vi "Monitoring task.vi"   [LabVIEW 2016]
types:
  T1 = cluster{bool, "测试模式":enum16{"水样测试", "平行样测试", "集成干预测试", "加标回收"}}
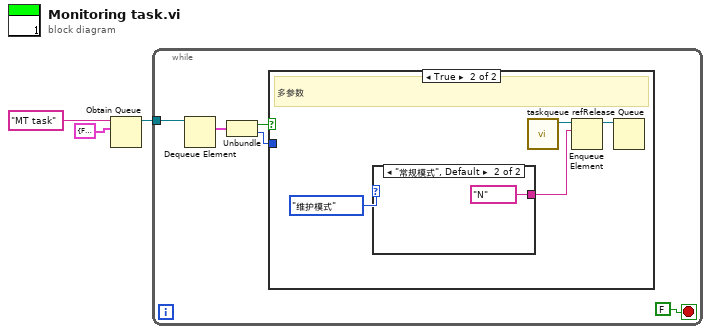
[diagram p0: block diagram]
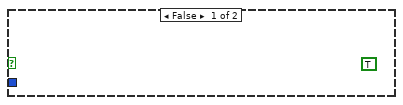
[diagram p2: hidden frame]
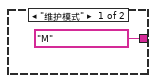
[diagram p3: hidden frame]
diagram:
  n1 = Obtain Queue(name (unnamed)="MT task" ("名称（未命名）"), element data type=T1 {FALSE, "测试模式"=enum."水样测试"}) -> (queue out=w2:refnum<queue>)  [unwired: 3 in, 2 out]
  n2 = while {
    tunnel: w2 -> [w8]
    stop <- FALSE stop-if-true
    n3 = Dequeue Element(queue=w8) -> (element=w6:T1)  [unwired: 2 in, 3 out]
    n4 = Unbundle(w6) -> (w5:bool, "测试模式"=w4:enum16{"水样测试", "平行样测试", "集成干预测试", "加标回收"})
    n5 = case shown="True" w5 {
      tunnel: w4 -> [_ _]
      frame False {
        (unwired) TRUE ("t")
      }
      frame True {
        # "多参数"
        n6 = case shown="\"常规模式\", Default" enum16{"维护模式", "常规模式", "应急模式", "质控模式"}."维护模式" ("运行模式") {
          tunnel: ["M" ("数据标记表") "N" ("数据标记表")] -> w12
          frame "维护模式" {
          }
          frame "常规模式", Default {
          }
        }
        n7 = call "taskqueue ref.vi"() -> ("队列输出"=w11:refnum<queue>)  [unwired: 10 in, 1 out]
        n8 = Enqueue Element(queue=w11, element=w12) -> (queue out=w10:refnum<queue>)  [unwired: 2 in, 2 out]
        n9 = Release Queue(queue=w10) -> ()  [unwired: 2 in, 3 out]
      }
    }
  }
